vi "String by Index.vi"(8 "error in (no error)":errorcluster, 10 "Index":i32, 11 "StringGroup in":refnum<class "Group STR.lvclass">) -> (0 "error out":errorcluster, 1 "Timestamp":dbl, 2 "String":string, 3 "StringGroup out":refnum<class "Group STR.lvclass">)   [LabVIEW 2020, in "Vecto.lvlib" / "Group STR.lvclass"]
uses:
  Group STR.lvclass
  Group STR.lvclass/Group STR.ctl
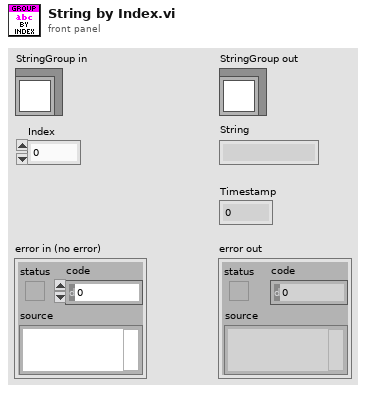
[diagram p1: front panel]
types:
  T1 = typedef "Vecto.lvlib/StringGroup.lvclass/Ref.ctl" = cluster{"Strings":string[], "Timestamp":dbl[]}
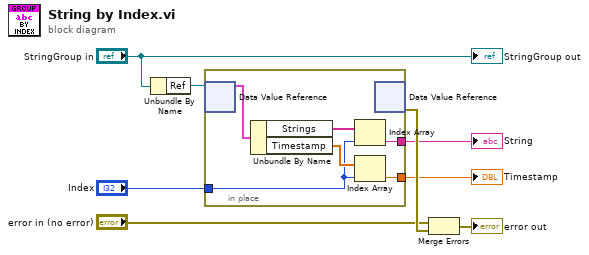
[diagram p0: block diagram]
diagram:
  n1 = Unbundle By Name("StringGroup in") -> ("Ref"=w6:refnum<data-value>)
  n2 = in-place {
    in-place-border: [w12] -> w4
    in-place-border: "Index" -> [w9]
    in-place-border: [w10] -> w1
    n3 = in-place-dvr #1(w6) -> (w14:T1)  [unwired: 1 out]
    n4 = Unbundle By Name(w14) -> ("Strings"=w13:string[], "Timestamp"=w11:dbl[])
    n5 = Index Array(array=w13, index=w9) -> (element=w12:string)
    n6 = Index Array(array=w11, index=w9) -> (element=w10:dbl)
    n7 = in-place-dvr #1() -> (w8:errorcluster)  [unwired: 1 in, 1 out]
  }
  "String" <- w4
  "Timestamp" <- w1
  n8 = Merge Errors("error in (no error)", w8) -> (→"error out":errorcluster)
  "StringGroup out" <- "StringGroup in"
